vi "Build Result Cluster.vi"(8 "error in (no error)":errorcluster, 9 "Pass?":bool, 10 "Actual Value":variant, 11 "Step in":refnum<class "Step.lvclass">) -> (0 "error out":errorcluster, 2 "Result":T1={"Step"="", "Actual Value"=variant, "Abort?"=FALSE, "Outcome"=enum."Skipped", "Error"={"status"=FALSE, "code"=0, "source"=""}}, 3 "Step out":refnum<class "Step.lvclass">)   [LabVIEW 2020, in "MacroAssert.lvlib" / "Step.lvclass"]
doc: "Builds a result cluster from the given step, <B>Actual Value</B>, and <B>Pass?</B>."
uses:
  Step.lvclass
  CTLs/Result.ctl
  CTLs/Outcome.ctl
  MacroAssert.lvlib
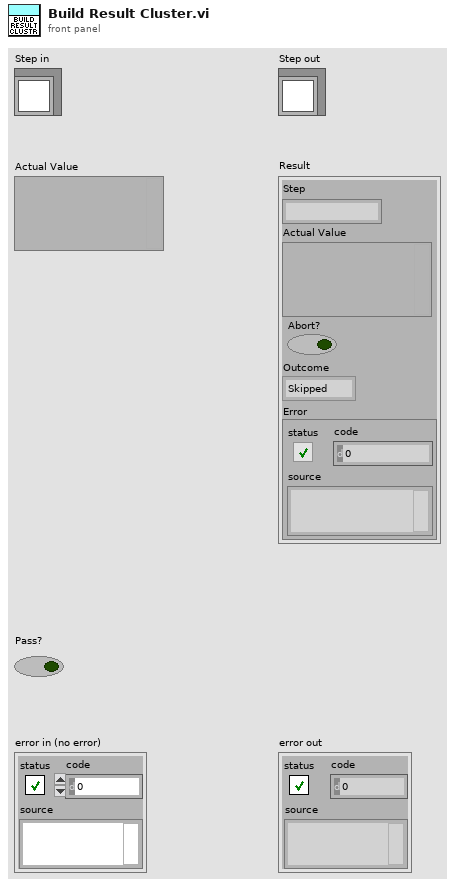
[diagram p1: front panel]
types:
  T1 = typedef "MacroAssert.lvlib/Result.ctl" = cluster{"Step":string, "Actual Value":variant, "Abort?":bool, "Outcome":T2, "Error":errorcluster}
  T2 = typedef "MacroAssert.lvlib/Outcome.ctl" = enum16{"Not Started", "Skipped", "Pass", "Fail", "Complete", "Error", "Auto Abort", "User Abort"}
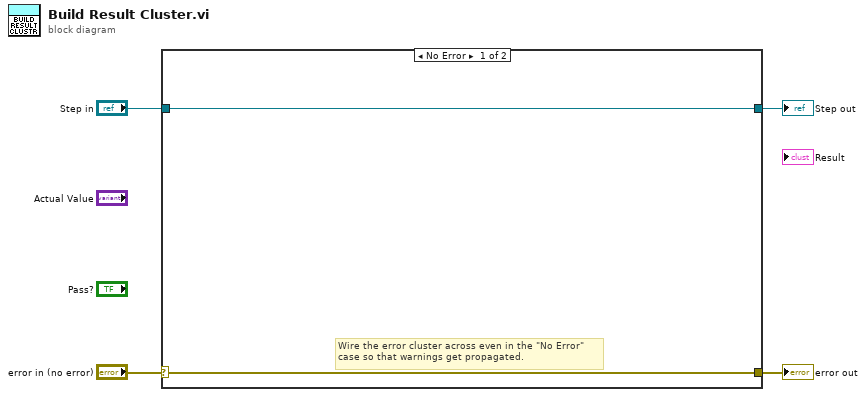
[diagram p0: block diagram]
diagram:
  n1 = case shown="No Error" "error in (no error)" {
    selector: "error in (no error)" -> [w5 w8]
    tunnel: [w5 w8] -> w3
    tunnel: [w6 w7] -> w1
    tunnel: "Step in" -> [w6 w7]
    frame No Error {
      # "Wire the error cluster across even in the \"No Error\"\ncase so that warnings get propagated."
    }
    frame Error {
    }
  }
  "error out" <- w3
  "Step out" <- w1
